vi "Close Progress Dialog.vi"(8 "error in (no error)":errorcluster, 11 "Progress Dialog in":refnum<class "Progress Dialog.lvclass">) -> (0 "error out":errorcluster)   [LabVIEW 2011, in "COSYLib.lvlib" / "Progress Dialog.lvclass"]
uses:
  Progress Dialog.lvclass
  Progress Dialog.lvclass/Progress Dialog.ctl
  COSYLib.lvlib
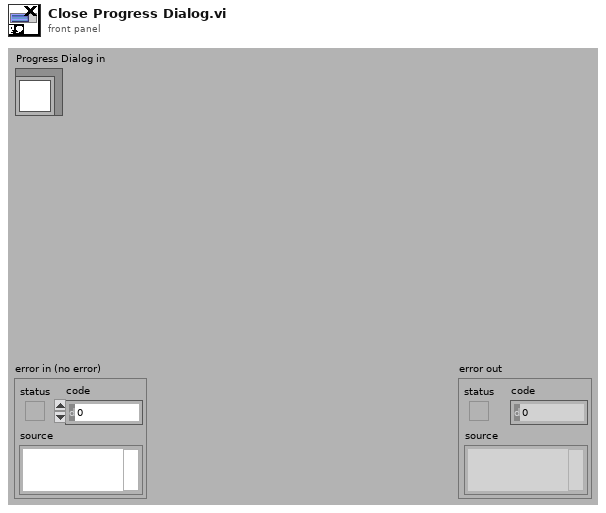
[diagram p1: front panel]
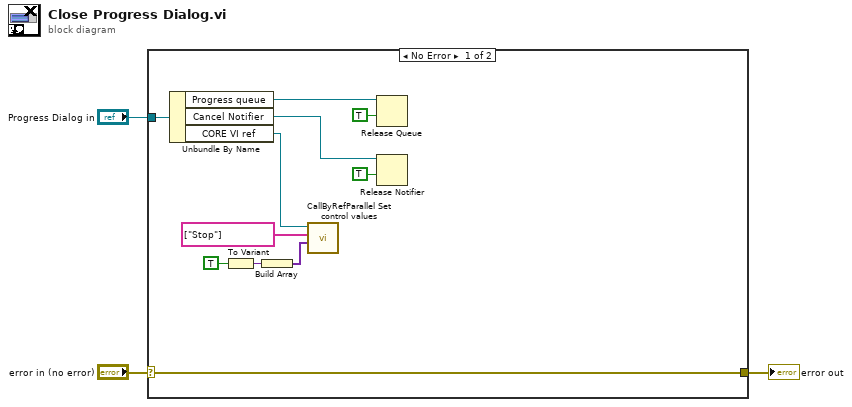
[diagram p0: block diagram]
diagram:
  n1 = case shown="No Error" "error in (no error)" {
    selector: "error in (no error)" -> [w14 w15]
    tunnel: [w14 w15] -> w2
    tunnel: "Progress Dialog in" -> [w13 _]
    frame No Error {
      n2 = Unbundle By Name(w13) -> ("Progress queue"=w12:refnum<queue>, "Cancel Notifier"=w11:refnum<notifier>, "CORE VI ref"=w8:refnum<vi>)
      n3 = To Variant(anything=TRUE) -> (Variant=w5:variant)
      n4 = Build Array(w5) -> (w4:variant[])
      n5 = call "CallByRefParallel Set control values.vi"("Control values"=w4, "Control names"=string[] ["Stop"], "VI Refnum"=w8) -> ()  [unwired: 7 in, 2 out]
      n6 = Release Queue(queue=w12, force destroy? (F)=TRUE) -> ()  [unwired: 1 in, 3 out]
      n7 = Release Notifier(notifier=w11, force destroy? (F)=TRUE) -> ()  [unwired: 1 in, 3 out]
    }
    frame Error {
    }
  }
  "error out" <- w2
